vi "Validate API Method (This Level).vi"(8 "error in (no error)":errorcluster, 10 "Command in":variant, 11 "Instrument in":refnum<class "Instrument.lvclass">) -> (0 "error out":errorcluster, 2 "command out":string, 3 "Instrument out":refnum<class "Instrument.lvclass">)   [LabVIEW 2019, in "Instrument.lvclass"]
uses:
  Instrument.lvclass
  <vilib>/Utility/Data Type/Get Numeric Information.vi
  105dbb1b-6b4f-4d0e-be68-45bd16370199.vi
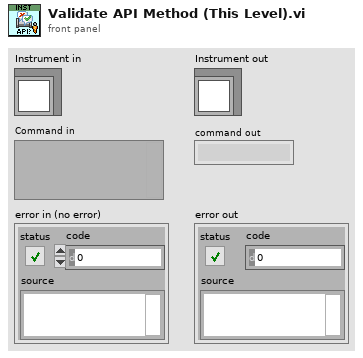
[diagram p1: front panel]
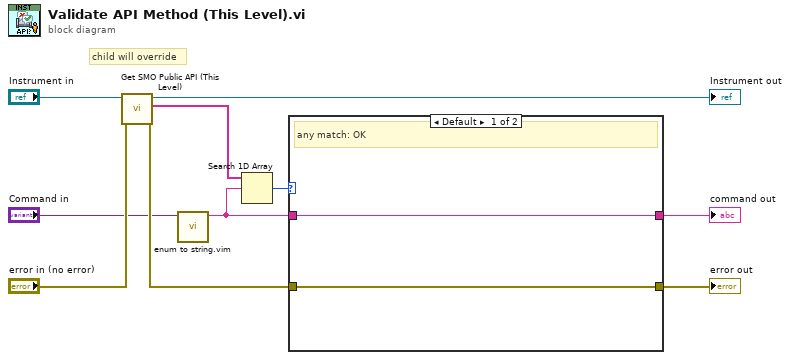
[diagram p0: block diagram]
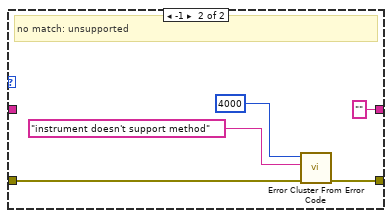
[diagram p2: hidden frame]
diagram:
  # "child will override"
  n1 = call-dynamic "Get SMO Public API (This Level).vi"("error in (no error)"="error in (no error)", "Instrument in"="Instrument in") -> ("error out"=w6:errorcluster, "commands (this level)"=w1:string[], "Instrument out"=→"Instrument out":refnum<class "Instrument.lvclass">)  [unwired: 7 in]
  n2 = call "enum to string.vim"("enum in"="Command in") -> ("string out"=w2:string)  [unwired: 9 in, 1 out]
  n3 = Search 1D Array(1D array=w1, element=w2) -> (index of element=w9:i32)  [unwired: 1 in]
  n4 = case shown="Default" w9 {
    tunnel: [w12 w15] -> w10
    tunnel: w6 -> [w12 w14]
    tunnel: [w11 "" ("command in")] -> w8
    tunnel: w2 -> [w11 _]
    frame Default {
      # "any match: OK"
    }
    frame -1 {
      # "no match: unsupported"
      n5 = call <vilib>:"Error Cluster From Error Code.vi"("error in (no error)"=w14, "error message (\"\")"="instrument doesn't support method" ("error message (\"\")"), "error code (0)"=4000) -> ("error out"=w15:errorcluster)  [unwired: 6 in]
    }
  }
  "error out" <- w10
  "command out" <- w8
